vi "VI Server_Close ONLY Controls Refs.vi"(8 "error in (no error)":errorcluster, 11 "VI Server Cluster":T1) -> (0 "error out":errorcluster)   [LabVIEW 2020, in "VI Server Toolkit LV2013.lvlib"]
doc: "<B>VI Server Cluster</B> contains targeted/called VI reference, array of controls/indicators labels and corresponding array of these controls generic references.\n\nThis VI closes <B>only control references</B> while VI reference kept open."
uses:
  VI Server Toolkit LV2013.lvlib
  VI Server_TypeDefs/VI Server_RefsCluster.ctl
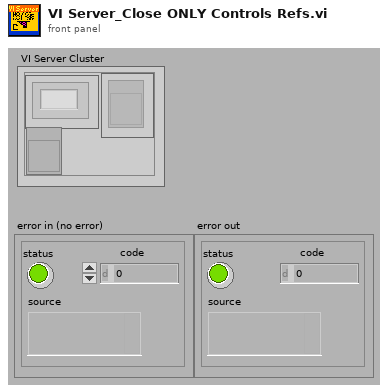
[diagram p1: front panel]
types:
  T1 = typedef "VI Server_RefsCluster.ctl" = cluster{"Labels":string[], "Refs":refnum<vi>[], "VI Ref":refnum<vi>}
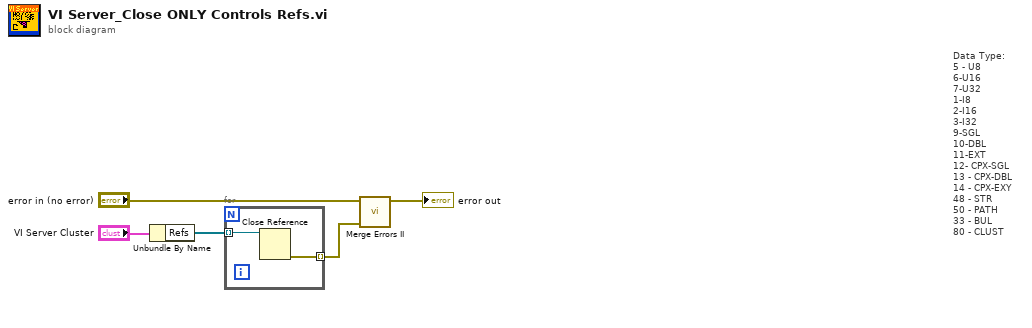
[diagram p0: block diagram]
diagram:
  # "Data Type:\n5 - U8\n6-U16\n7-U32\n1-I8\n2-I16\n3-I32\n9-SGL\n10-DBL\n11-EXT\n12- CPX-SGL\n13 - CPX-DBL\n14 - CPX-EXY\n48 - STR\n50 - PATH\n33 - BUL\n80 - CLUST"
  n1 = Unbundle By Name("VI Server Cluster") -> ("Refs"=w4:refnum<vi>[])
  n2 = for {
    tunnel: w4 -> [w7] mode=indexing
    tunnel: [w6] -> w3 mode=indexing
    n3 = Close Reference(reference=w7) -> (error out=w6:errorcluster)  [unwired: 1 in]
  }
  n4 = call "Merge Errors II.vi"("error array in"=w3, "error in 1 (no error)"="error in (no error)") -> ("error out.DUP"=→"error out":errorcluster)  [unwired: 2 in, 3 out]
